vi "Solution part 2a.vi"(11 "data?":bool) -> ()   [LabVIEW 2020]
panel:
  out "sorted array":cluster{"bus id":i32, "index":i32}[](array[cluster])
  out "loop index":u64
  out "max bus ID":cluster{"bus id":i32, "index":i32}
  in  "manual input":string
  in  "file input?":bool
  out "Timestamp":u64
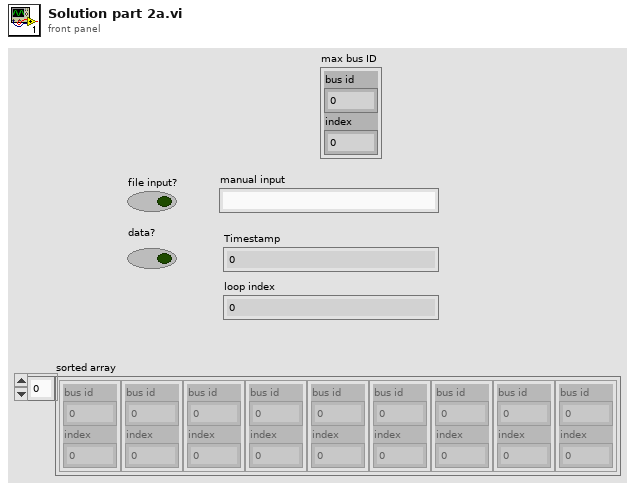
[diagram p1: front panel]
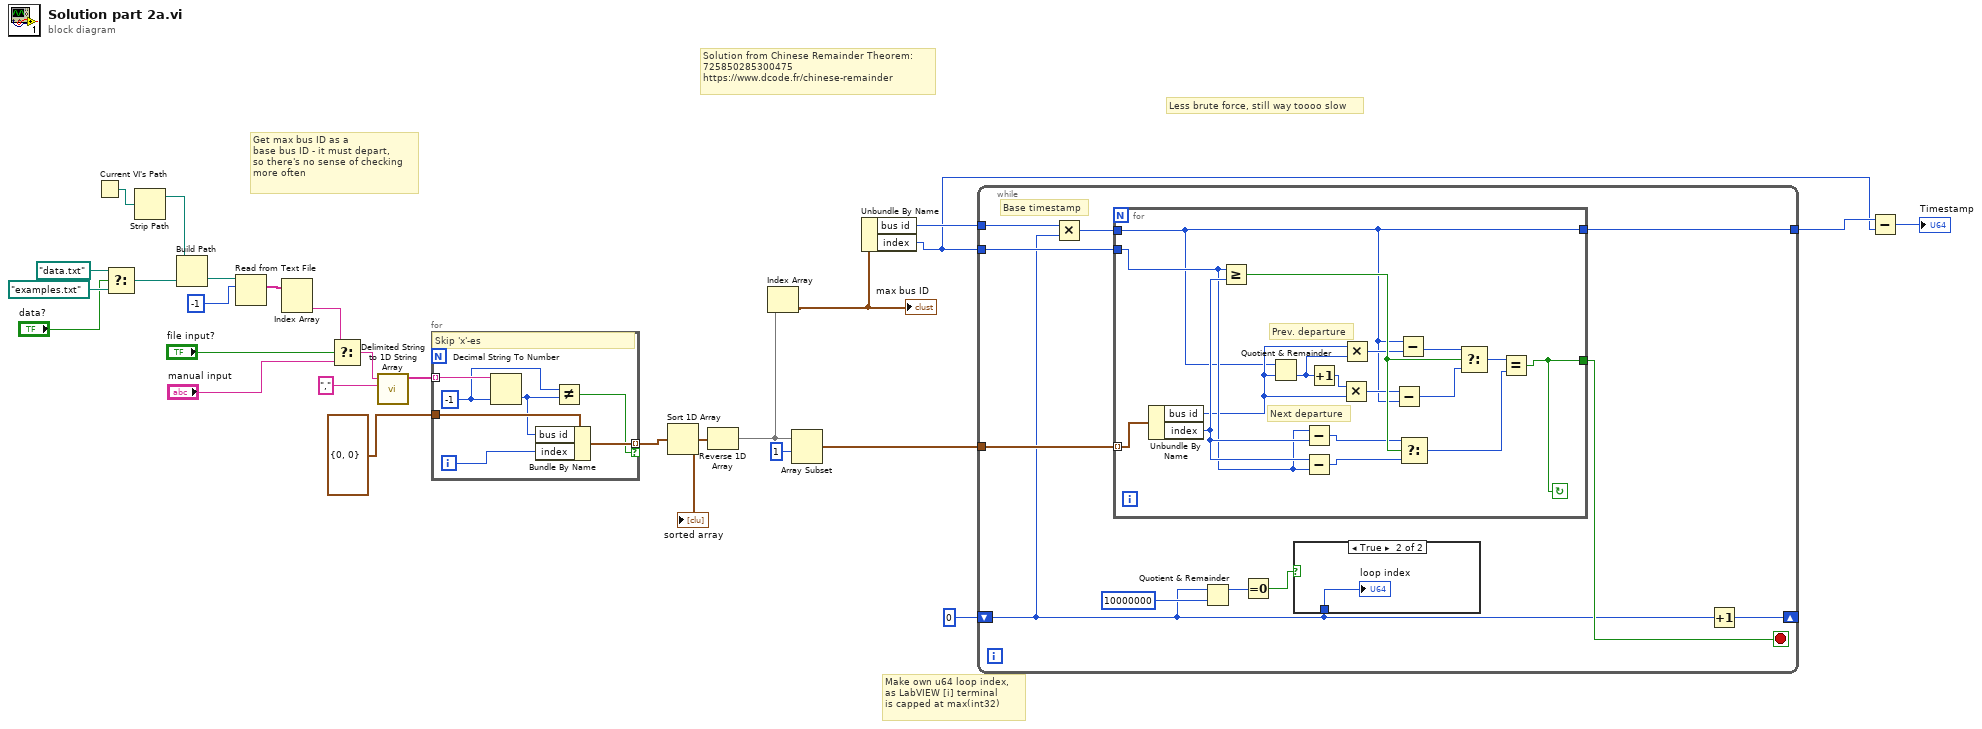
[diagram p0: block diagram]
diagram:
  # "Solution from Chinese Remainder Theorem:\n725850285300475\nhttps://www.dcode.fr/chinese-remainder"
  # "Less brute force, still way toooo slow"
  # "Make own u64 loop index,\nas LabVIEW [i] terminal\nis capped at max(int32)"
  # "Get max bus ID as a\nbase bus ID - it must depart,\nso there's no sense of checking\nmore often"
  n1 = Current VI's Path() -> (path=w24:path)
  n2 = Select(t=path "data.txt", s="data?", f=path "examples.txt") -> (s? t:f=w25:path)
  n3 = Strip Path(path=w24) -> (stripped path=w23:path)  [unwired: 1 out]
  n4 = Build Path(base path=w23, name or relative path=w25) -> (appended path=w22:path)
  n5 = Read from Text File(file (use dialog)=w22, count=-1) -> (text=w19:string[])  [unwired: 2 in, 3 out]
  n6 = Index Array(array=w19) -> (element #2=w18:string)  [unwired: 2 in, 1 out]
  n7 = Select(t=w18, s="file input?", f="manual input") -> (s? t:f=w16:string)
  n8 = call <vilib>:"Delimited String to 1D String Array.vi"("delimiter"=",", "delimited string"=w16) -> ("string array"=w13:string[])  [unwired: 9 in]
  n9 = for {
    tunnel: w13 -> [w34] mode=indexing
    tunnel: cluster{"bus id":i32, "index":i32} {"bus id"=0, "index"=0} -> [w33]
    tunnel: [w31] -> w4 mode=indexing if=w28
    i -> [w32]
    w29 = -1 ("default (0 I32)")
    # "Skip 'x'-es"
    n10 = Decimal String To Number(string=w34, default (0L)=w29) -> (number=w30:i32)  [unwired: 1 in, 1 out]
    n11 = Bundle By Name(cluster=w33, "bus id"=w30, "index"=w32) -> (w31:cluster{"bus id":i32, "index":i32})
    n12 = Not Equal?(x=w29, y=w30) -> (x != y?=w28:bool)
  }
  n13 = Sort 1D Array(array=w4) -> (sorted array=w9:cluster{"bus id":i32, "index":i32}[])
  "sorted array" <- w9
  n14 = Reverse 1D Array(array=w9) -> (reversed array=w7:cluster{"bus id":i32, "index":i32}[])
  n15 = Index Array(array=w7) -> (element=w8:cluster{"bus id":i32, "index":i32})  [unwired: 1 in]
  "max bus ID" <- w8
  n16 = Array Subset(array=w7, index=1) -> (w5:cluster{"bus id":i32, "index":i32}[])  [unwired: 1 in]
  n17 = Unbundle By Name(w8) -> ("bus id"=w10:i32, "index"=w2:i32)
  n18 = while {
    tunnel: w10 -> [w44]
    shift-right: [w45] -> _
    shift-left: u64 0 ("index") -> [w35]
    tunnel: w5 -> [w41]
    tunnel: w2 -> [w40]
    tunnel: [w39] -> w3
    stop <- w42 stop-if-true
    # "Base timestamp"
    n19 = Multiply(x=w44, y=w35) -> (x*y=w43:u64)
    n20 = for {
      tunnel: [w63] -> w42
      tunnel: w43 -> [w47]
      tunnel: w41 -> [w61] mode=indexing
      tunnel: w40 -> [w55]
      tunnel: [w47] -> w39
      stop <- w63 continue-if-true
      # "Next departure"
      # "Prev. departure"
      n21 = Unbundle By Name(w61) -> ("bus id"=w49:i32, "index"=w56:i32)
      n22 = Greater Or Equal?(x=w55, y=w56) -> (x >= y?=w60:bool)
      n23 = Quotient & Remainder(x=w47, y=w49) -> (floor(x/y)=w50:u64)  [unwired: 1 out]
      n24 = Subtract(x=w55, y=w56) -> (x-y=w59:i32)
      n25 = Subtract(x=w56, y=w55) -> (x-y=w58:i32)
      n26 = Increment(x=w50) -> (x+1=w62:u64)
      n27 = Multiply(x=w62, y=w49) -> (x*y=w51:u64)
      n28 = Multiply(x=w49, y=w50) -> (x*y=w48:u64)
      n29 = Subtract(x=w51, y=w47) -> (x-y=w54:u64)
      n30 = Subtract(x=w47, y=w48) -> (x-y=w53:u64)
      n31 = Select(t=w59, s=w60, f=w58) -> (s? t:f=w57:i32)
      n32 = Select(t=w53, s=w60, f=w54) -> (s? t:f=w52:u64)
      n33 = Equal?(x=w52, y=w57) -> (x = y?=w63:bool)
    }
    n34 = Quotient & Remainder(x=w35, y=u64 10000000) -> (x-y*floor(x/y)=w37:u64)  [unwired: 1 out]
    n35 = Equal To 0?(x=w37) -> (x = 0?=w36:bool)
    n36 = case shown="True" w36 {
      tunnel: w35 -> [_ w46]
      frame False {
      }
      frame True {
        "loop index" <- w46
      }
    }
    n37 = Increment(x=w35) -> (x+1=w45:u64)
  }
  n38 = Subtract(x=w3, y=w2) -> (x-y=→"Timestamp":u64)
